vi "ProtobufDoubleAnalogWaveformToLVAnalogWaveform.vi"(8 "error in (no error)":errorcluster, 11 "ni_protobuf_types_DoubleAnalogWaveform_Flat":T1) -> (0 "error out":errorcluster, 3 "Waveform":waveform(dbl))   [LabVIEW 2020, in "Extensions.lvlib"]
uses:
  <vilib>/gRPC/Extensions/Extensions.lvlib
  <vilib>/gRPC/Generated APIs/ni/protobuf/types/RPC Messages/ni_protobuf_types_DoubleAnalogWaveform_Flat.ctl
  <vilib>/gRPC/Generated APIs/ni/protobuf/types/RPC Messages/ni_protobuf_types_PrecisionTimestamp_Flat.ctl
  <vilib>/gRPC/Generated APIs/ni/protobuf/types/RPC Messages/ni_protobuf_types_DoubleAnalogWaveform_AttributesEntry_Flat.ctl
  <vilib>/gRPC/Generated APIs/ni/protobuf/types/RPC Messages/ni_protobuf_types_WaveformAttributeValue_Flat.ctl
  <vilib>/gRPC/Generated APIs/ni/protobuf/types/ni.protobuf.types.lvlib
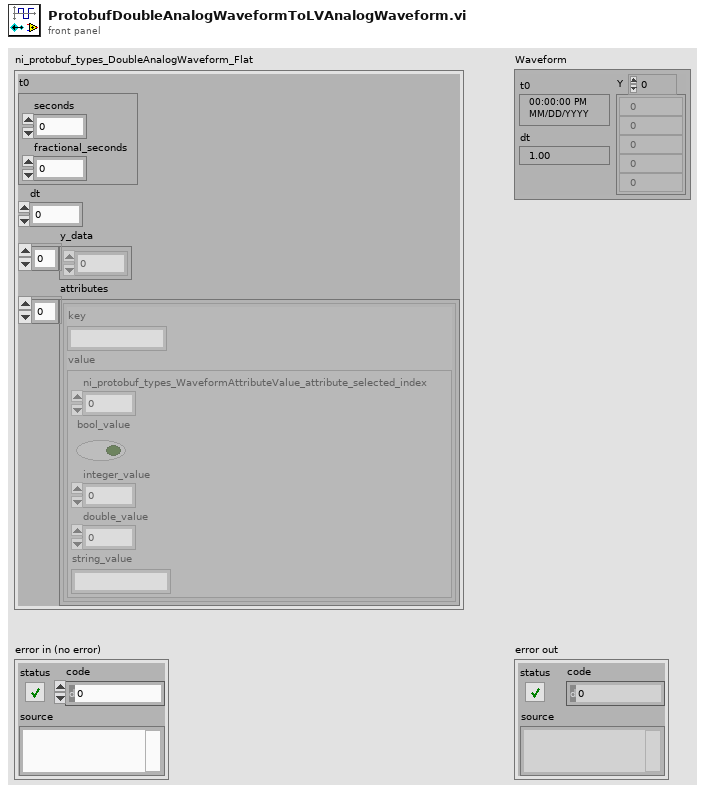
[diagram p1: front panel]
types:
  T1 = typedef "ni.protobuf.types.lvlib/ni_protobuf_types_DoubleAnalogWaveform_Flat.ctl" = cluster{"t0":T2, "dt":dbl, "y_data":dbl[], "attributes":T3[]}
  T2 = typedef "ni.protobuf.types.lvlib/ni_protobuf_types_PrecisionTimestamp_Flat.ctl" = cluster{"seconds":i64, "fractional_seconds":u64}
  T3 = typedef "ni.protobuf.types.lvlib/ni_protobuf_types_DoubleAnalogWaveform_AttributesEntry_Flat.ctl" = cluster{"key":string, "value":T4}
  T4 = typedef "ni.protobuf.types.lvlib/ni_protobuf_types_WaveformAttributeValue_Flat.ctl" = cluster{"ni_protobuf_types_WaveformAttributeValue_attribute_selected_index":i32, "bool_value":bool, "integer_value":i32, "double_value":dbl, "string_value":string}
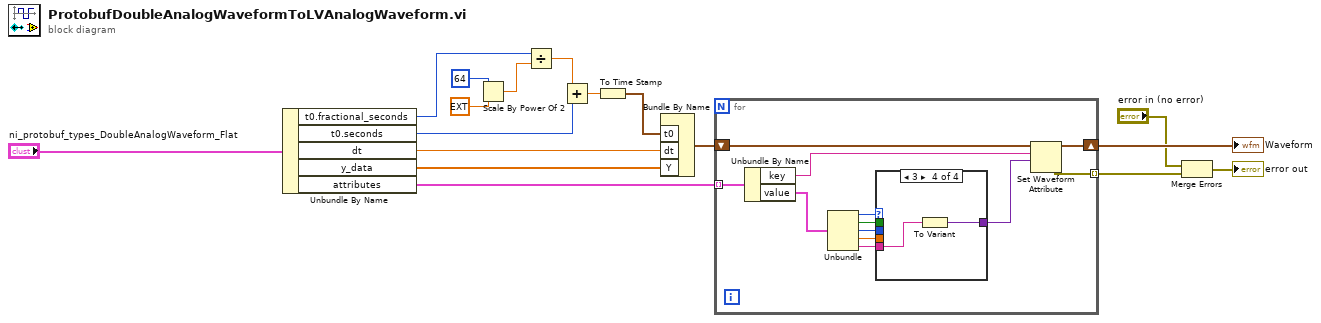
[diagram p0: block diagram]
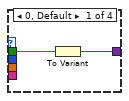
[diagram p2: hidden frame]
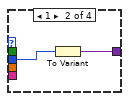
[diagram p3: hidden frame]
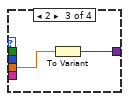
[diagram p4: hidden frame]
diagram:
  n1 = Unbundle By Name("ni_protobuf_types_DoubleAnalogWaveform_Flat") -> ("t0.fractional_seconds"=w14:u64, "t0.seconds"=w11:i64, "dt"=w8:dbl, "y_data"=w7:dbl[], "attributes"=w6:T3[])
  n2 = Scale By Power Of 2(n=i16 64, x=ext 1.0) -> (x*2^n=w13:ext)
  n3 = Divide(x=w14, y=w13) -> (x/y=w12:ext)
  n4 = Add(x=w12, y=w11) -> (x+y=w10:ext)
  n5 = To Time Stamp(1:w10) -> (0:w9:timestamp)
  n6 = Bundle By Name("t0"=w9, "dt"=w8, "Y"=w7) -> (w5:waveform(dbl))  [unwired: 1 in]
  n7 = for {
    tunnel: w6 -> [w29] mode=indexing
    shift-right: [w25] -> w4
    shift-left: w5 -> [w27]
    tunnel: [w18] -> w3 mode=indexing
    n8 = Unbundle By Name(w29) -> ("key"=w28:string, "value"=w26:T4)
    n9 = Unbundle(w26) -> ("ni_protobuf_types_WaveformAttributeValue_attribute_selected_index"=w24:i32, "bool_value"=w23:bool, "integer_value"=w21:i32, "double_value"=w20:dbl, "string_value"=w19:string)
    n10 = case shown="3" w24 {
      tunnel: w23 -> [w31 _ _ _]
      tunnel: [w30 w33 w35 w37] -> w22
      tunnel: w21 -> [_ w32 _ _]
      tunnel: w20 -> [_ _ w34 _]
      tunnel: w19 -> [_ _ _ w36]
      frame 0, Default {
        n11 = To Variant(anything=w31) -> (Variant=w30:variant)
      }
      frame 1 {
        n12 = To Variant(anything=w32) -> (Variant=w33:variant)
      }
      frame 2 {
        n13 = To Variant(anything=w34) -> (Variant=w35:variant)
      }
      frame 3 {
        n14 = To Variant(anything=w36) -> (Variant=w37:variant)
      }
    }
    n15 = Set Waveform Attribute(5:w22, 6:w28, 7:w27) -> (0:w18:errorcluster, 3:w25:waveform(dbl))  [unwired: 1 in, 1 out]
  }
  "Waveform" <- w4
  n16 = Merge Errors("error in (no error)", w3) -> (→"error out":errorcluster)
